vi "GetSupportedMetrics.vi"(11 "key values":T1[](array[typedef])) -> (3 "supported metrics":string[](array[string]))   [LabVIEW 2017, in "GlobalConfiguration.lvlib"]
uses:
  <vilib>/addons/InsightCM/Utilities/GlobalConfiguration/GlobalConfiguration.lvlib
  <vilib>/addons/InsightCM/MessageBus/Base/controls/SectionKeyValues.ctl
  <vilib>/addons/InsightCM/MessageBus/Base/controls/KeyValuePair.ctl
  <vilib>/addons/InsightCM/Utilities/Analysis/Shared/AnalysisHelper.lvlib
  <vilib>/addons/InsightCM/Utilities/PropertyHelpers/PropertyHelpers.lvlib
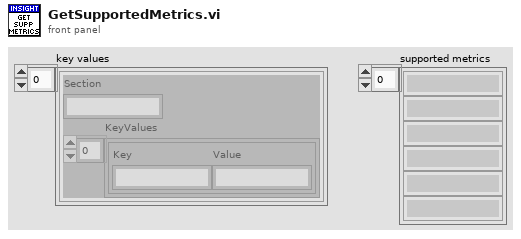
[diagram p1: front panel]
types:
  T1 = typedef "SectionKeyValues.ctl" = cluster{"Section":string, "KeyValues":T2[]}
  T2 = typedef "KeyValuePair.ctl" = cluster{"Key":string, "Value":string}
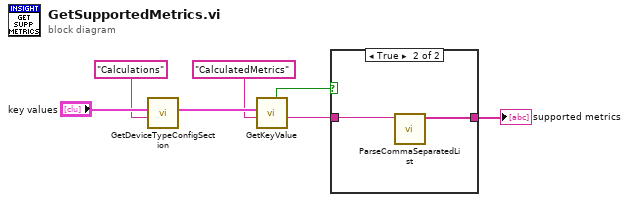
[diagram p0: block diagram]
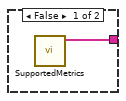
[diagram p2: hidden frame]
diagram:
  n1 = call <vilib>:"GetDeviceTypeConfigSection.vi"("key"="Calculations", "key values"="key values") -> ("key value pairs out"=w5:T2[])  [unwired: 8 in, 1 out]
  n2 = call <vilib>:"GetKeyValue.vi"("key"="CalculatedMetrics", "key value pairs"=w5) -> ("value"=w2:string, "found"=w1:bool)  [unwired: 7 in, 1 out]
  n3 = case shown="True" w1 {
    tunnel: [w8 w9] -> w3
    tunnel: w2 -> [_ w10]
    frame False {
      n4 = call <vilib>:"SupportedMetrics.vi"() -> ("Supported Metrics"=w8:string[])  [unwired: 11 in]
    }
    frame True {
      n5 = call <vilib>:"ParseCommaSeparatedList.vi"("List"=w10) -> ("Array"=w9:string[])  [unwired: 10 in]
    }
  }
  "supported metrics" <- w3
